vi "SendCommand.vi"(0 "Propeller":i32, 1 "error in (no error)":errorcluster, 2 "NXTObject":T1 {"nxtIterHandle" format="%08x"; "modIterHandle" format="%08x"; "moduleHandle" format="%08x"; "fileIterHandle" format="%08x"; "fileHandle" format="%08x"; "nxtHandle" format="%08x"}, 3 "Procedure":i32, 5 "Rudder":i32) -> (4 "error out":errorcluster)   [LabVIEW 2011]
uses:
  <vilib>/NXT/Block Support/nxt.ctl
panel:
  out "NXTCommand":string
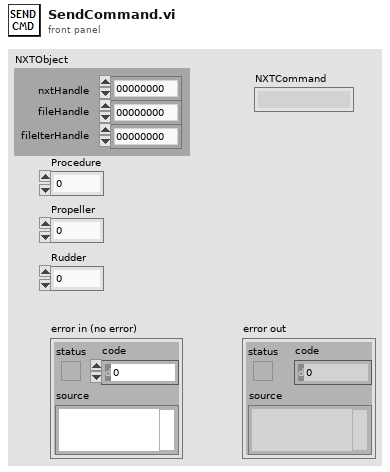
[diagram p1: front panel]
types:
  T1 = typedef "nxt.ctl" = cluster{"nxtHandle":u32, "fileHandle":u32, "fileIterHandle":u32, "moduleHandle":u32, "modIterHandle":u32, "nxtIterHandle":u32}
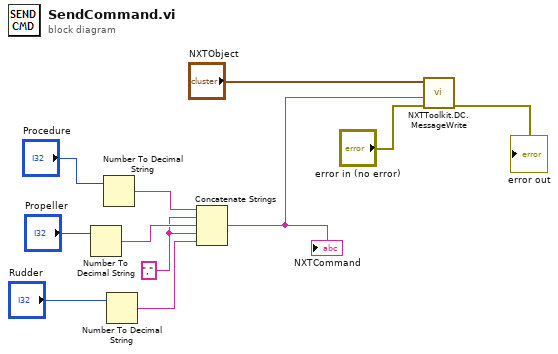
[diagram p0: block diagram]
diagram:
  w7 = "," ("string")
  n1 = Number To Decimal String ("Propeller")(number="Propeller") -> (decimal integer string=w10:string)  [unwired: 1 in]
  n2 = Number To Decimal String ("Procedure")(number="Procedure") -> (decimal integer string=w8:string)  [unwired: 1 in]
  n3 = Number To Decimal String ("Rudder")(number="Rudder") -> (decimal integer string=w9:string)  [unwired: 1 in]
  n4 = Concatenate Strings(w8, w7, w10, w7, w9) -> (w6:string)
  "NXTCommand" <- w6
  n5 = call <vilib>:"NXTToolkit.DC.MessageWrite.vi"("error in (no error)"="error in (no error)", "Message"=w6, "NXTObject"="NXTObject") -> ("error out"=→"error out":errorcluster)  [unwired: 5 in, 3 out]
